vi "TransformHelper.vi"(8 "error in (no error)":errorcluster, 9 "Multiplier":sgl, 10 "Power":sgl, 11 "Image  in":T1) -> (0 "error out":errorcluster, 1 "Time, ms":u32, 3 "Image out":T1)   [LabVIEW 2023]
uses:
  <vilib>/vision/Image Controls.llb/IMAQ Image.ctl
  MP Helper.dll
panel:
  in  "Divider":dbl=100.0 format="%#_13g"
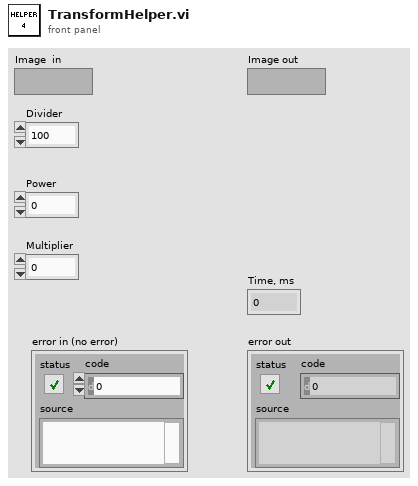
[diagram p1: front panel]
types:
  T1 = typedef "IMAQ Image.ctl" = refnum<image>
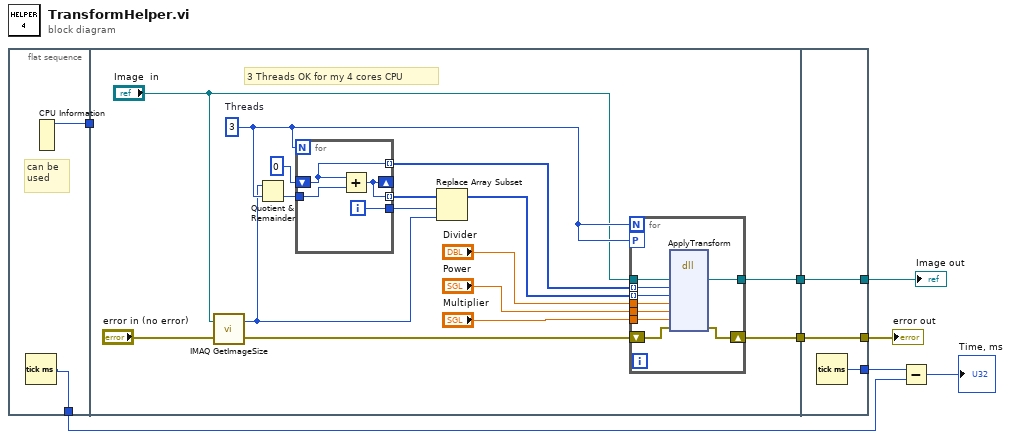
[diagram p0: block diagram]
diagram:
  n1 = flat-sequence {
    tunnel: [w10] -> w2
    tunnel: [w9] -> w1
    tunnel: [w21] -> w5
    tunnel: [w14] -> w3
    tunnel: w1 -> [_]
    tunnel: [w42] -> w8
    tunnel: [w41] -> w6
    tunnel: w5 -> [w41]
    tunnel: [w40] -> w4
    tunnel: w3 -> [w40]
    frame #0 {
      # "can be\nused"
      n2 = Tick Count (ms)() -> (millisecond timer value=w10:u32)
      n3 = CPU Information() -> (4:w9:i32)  [unwired: 3 out]
    }
    frame #1 {
      w13 = 3  # Threads
      # "3 Threads OK for my 4 cores CPU"
      n4 = call "IMAQ GetImageSize"("Image"="Image  in", "error in (no error)"="error in (no error)") -> ("Y Resolution"=w11:i32, "error out"=w22:errorcluster)  [unwired: 2 in, 1 out]
      n5 = Quotient & Remainder(x=w11, y=w13) -> (floor(x/y)=w20:i32)  [unwired: 1 out]
      n6 = for {
        N: w13 -> [_]
        tunnel: w20 -> [w39]
        shift-right: [w37] -> _
        shift-left: 0 -> [w38]
        tunnel: [w38] -> w16 mode=indexing
        tunnel: [w37] -> w18 mode=indexing
        tunnel: [w36] -> w17
        i -> [w36]
        n7 = Add(x=w38, y=w39) -> (x+y=w37:i32)
      }
      n8 = Replace Array Subset(array=w18, new element=w11, index=w17) -> (w15:i32[])
      n9 = for {
        N: w13 -> [_]
        tunnel: "Divider" -> [w35]
        tunnel: "Power" -> [w34]
        tunnel: "Multiplier" -> [w33]
        tunnel: w16 -> [w32] mode=indexing
        tunnel: [w30] -> w21
        tunnel: w15 -> [w28] mode=indexing
        shift-right: [w29] -> w14
        shift-left: w22 -> [w31]
        workers-P: w13 -> [_]
        tunnel: "Image  in" -> [w27]
        n10 = dll-call lib="C:/Users/Andrey/Desktop/xe1clean2/HelperDLL/MP Helper.dll" fn="ApplyTransform"(w27, "StartLine"=w32, "EndLine"=w28, "Divider"=w35, "Power"=w34, "Multiplier"=w33, "arg5"=w31) -> (w30:T1, "arg5"=w29:errorcluster)  [unwired: 9 in, 2 out]
      }
    }
    frame #2 {
      n11 = Tick Count (ms)() -> (millisecond timer value=w42:u32)
    }
  }
  n12 = Subtract(x=w8, y=w2) -> (x-y=→"Time, ms":u32)
  "Image out" <- w6
  "error out" <- w4
